vi "manual_action.vi"(7 "references":T1, 8 "error in (no error)":errorcluster, 10 "data":variant, 11 "step":string) -> (0 "error out":errorcluster)   [LabVIEW 2015, in "repub-dvr_nre.lvlib"]
uses:
  repub-dvr_nre.lvlib
  _controls/references.ctl
  private/_controls/input.ctl
  private/_controls/input_command.ctl
  private/_controls/output.ctl
  private/_controls/data.ctl
  _controls/configuration.ctl
  lv-recipe-machine/private/_controls/recipe_data.ctl
  lv-recipe-machine/public/_controls/mode.ctl
  lv-recipe-machine/public/_controls/manual_state.ctl
  lv-recipe-machine/public/_controls/automatic_state.ctl
  <userlib>/antonio-alexander/lv-waitgroup/public/_controls/api_waitgroup.ctl
  lv-recipe-machine/public/_controls/transition.ctl
  _controls/change.ctl
  _controls/status.ctl
  lv-recipe-machine/lv-recipe-machine.lvlib
  <userlib>/antonio-alexander/lv-waitgroup/lv-waitgroup.lvlib
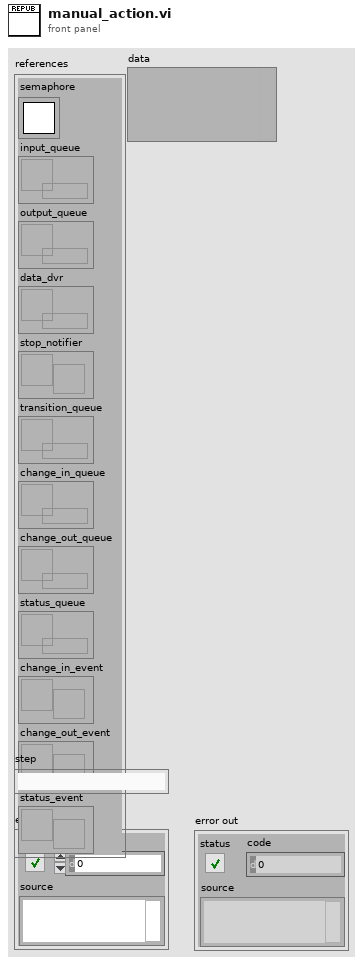
[diagram p1: front panel]
types:
  T1 = typedef "repub-dvr_nre.lvlib/references.ctl" = cluster{"semaphore":T2, "input_queue":refnum<queue>, "output_queue":refnum<queue>, "data_dvr":refnum<data-value>, "stop_notifier":refnum<notifier>, "transition_queue":refnum<queue>, "change_in_queue":refnum<queue>, "change_out_queue":refnum<queue>, "status_queue":refnum<queue>, "change_in_event":refnum<user-event>, "change_out_event":refnum<user-event>, "status_event":refnum<user-event>}
  T2 = typedef "Semaphore RefNum" = refnum<k1>
  T3 = typedef "lv-recipe-machine.lvlib/manual_state.ctl" = enum16{"<manual_state>", "failed", "action", "running", "idle", "<null>"}
  T4 = typedef "repub-dvr_nre.lvlib/data.ctl" = cluster{"configuration":T5, "working":cluster{"recipe_data":T6, "api_waitgroup":T9}}
  T5 = typedef "repub-dvr_nre.lvlib/configuration.ctl" = cluster{dbl}
  T6 = typedef "lv-recipe-machine.lvlib/recipe_data.ctl" = cluster{"mode":T7, "manual_state":T3, "automatic_state":T8, "step":string, "automatic_recipe":variant, "manual_actions":variant, "manual_data":variant, "automatic_data":variant}
  T7 = typedef "lv-recipe-machine.lvlib/mode.ctl" = enum16{"<mode>", "manual", "automatic", "<null>"}
  T8 = typedef "lv-recipe-machine.lvlib/automatic_state.ctl" = enum16{"<automatic_state>", "failed", "idle", "running", "paused", "transition", "stopped", "<null>"}
  T9 = typedef "lv-waitgroup.lvlib/api_waitgroup.ctl" = cluster{"waitgroups":refnum<data-value>, "waitgroup":string}
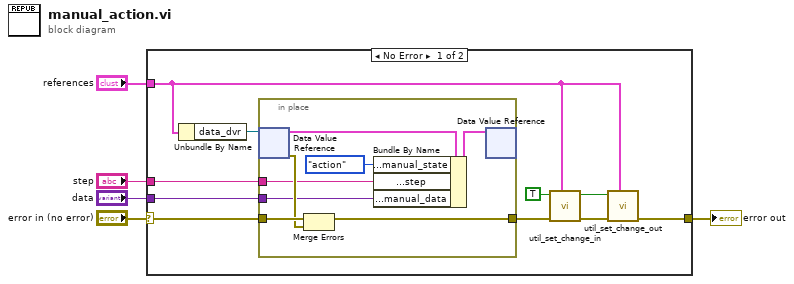
[diagram p0: block diagram]
diagram:
  n1 = case shown="No Error" "error in (no error)" {
    selector: "error in (no error)" -> [w13 w23]
    tunnel: [w9 w23] -> w4
    tunnel: "references" -> [w8 _]
    tunnel: "step" -> [w12 _]
    tunnel: "data" -> [w6 _]
    frame No Error {
      w7 = TRUE ("change")
      n2 = Unbundle By Name(w8) -> ("data_dvr"=w14:refnum<data-value>)
      n3 = in-place {
        in-place-border: [w20] -> w11
        in-place-border: w13 -> [w22]
        in-place-border: w12 -> [w16]
        in-place-border: w6 -> [w15]
        n4 = in-place-dvr #1(w14) -> (w19:T4, w21:errorcluster)
        n5 = Merge Errors(w22, w21) -> (w20:errorcluster)
        n6 = Bundle By Name(cluster=w19, "working.recipe_data.manual_state"=manual_state."action", "working.recipe_data.step"=w16, "working.recipe_data.manual_data"=w15) -> (w18:T4)
        n7 = in-place-dvr #1(w18) -> ()  [unwired: 2 out]
      }
      n8 = call "util_set_change_in.vi"("references"=w8, "error in (no error)"=w11, "change"=w7) -> ("error out"=w10:errorcluster)  [unwired: 8 in]
      n9 = call "util_set_change_out.vi"("references"=w8, "error in (no error)"=w10, "change"=w7) -> ("error out"=w9:errorcluster)  [unwired: 8 in]
    }
    frame Error {
    }
  }
  "error out" <- w4
